vi "Generate Oximetry Plots-Rev1.vi"(10 "Spectral Data":T1={"PDT Amp [v]"=0.0, "RIS Amp [v]"=0.0, "B-Field"=[], "All In-Phase Scan Spectra"=[], "Model Select"=enum."OneCompRISTwoPDT", "Fit Each Scan"=FALSE, "PDT Center [g]"=0.0, "In-Phase Average Spectra"=[], "In-Phase Median Spectra"=[], "Out-Phase Median Spectra"=[], "Out-Phase Average Spectra"=[], "Fit Spectra"=[], "Fit No-Baseline Spectra"=[], "All Out-Phase Scan Spectra"=[], "Baseline Offset Correction"=FALSE, "In-Phase Offset [v]"=0.0, "Out-Phase Offset [v]"=0.0, "Ch2 Input\n(Balance)"=[], "Ch3 Input\n(Phase)"=[], "Ch4 Input\n(AFC)"=[], "Fit Pars"=[], "Fit Pars Errors"=[], "Fit Pars Labels"=[], "Raw Scan DAQ Data"=[], "Bad Scans Indicies"=[], "Good In-Phase Scan Spectra"=[], "Good Out-Phase Scan Spectra"=[], "Bad In-Phase Scan Spectra"=[], "Bad Out-Phase Scan Spectra"=[], "Number of bad scans"=0, "Fit History"=[], "PDT Amp. History/Set [v]"=[], "RIS Amp. History/Set [v]"=[], "RIS Amp. History/Scan [v]"=[], "All Shifted B-Fields"=[], "Good Shifted B-Fields"=[], "Ch5 Input\n(SpO2)"=[], "Ch6 Input\n(BPM)"=[], "Global SNR"=0.0, "Fit Error History"=[], "SNR History"=[]} {"Global SNR" min=0.0; "PDT Center [g]" min=0.0; "RIS Amp [v]" min=0.0; "PDT Amp [v]" min=0.0}, 11 "Measurement Information":T3={"Comments"="", "Directory Input"="", "Data file path"=path "C:/Data/EPR Data", "Scripting File"=path "C:/Data/Configuration Script.csv", "Save Data"=FALSE, "Tooth size (d11) [mm]"=0.0, "Tooth size (d12) [mm]"=0.0, "Tooth size (d21) [mm]"=0.0, "Tooth size (d22) [mm]"=0.0, "Dose of Tooth [Gy]"=0.0, "Safe Shutdown?"=FALSE, "Gases Available"=[], "Database Username"="", "Database Password"="", "Database Login URL"="", "Database Upload URL"="", "Database Success URL"="", "Database XML URL"="", "Database Resonator URL"="", "Session Number"=0, "Set #"=1, "Resonator Operator"="", "Session Type"="", "Tooth/Sample ID"="", "Volunteer ID"="", "Computer Operator"="", "Volunteer Type"="", "Site/Tooth Selection (T8,T9)"="", "Resonator"="", "Measurement Site"="", "Non-standard session?"=FALSE, "EPR DAQ Version"="", "Session Path"=path "C:/Data/EPR Data", "Chosen Applied State"="", "Chosen Initial State"="", "Time of Transition"="", "DAQ Mode"=enum."Engineering", "pO2/Scan [mmHg]"=[], "pO2/Set [mmHg]"=[], "Linewidth (HWHM)/Scan [Gauss]"=[], "Linewidth (HWHM)/Set [Gauss]"=[], "pO2 Conversion"="", "Dose Calibration Cluster"={"Dose Response"={"grand_mean"=0.0292016, "slope"=0.0188720543}, "Dose Correction"={"Sex"=1, "a0"=7.719669421, "a1"=-2.746550736, "a2"=-0.186490355, "a3"=0.041922063, "a4"=-0.849147359, "a5"=0.14330063, "a6"=0.019930219, "A_n"=40.0, "H_n"=10.12, "Dose Correction"=FALSE}, "Dose Reporting"={"Reporting is"=TRUE, "sd_threshold [AU]"=0.06, "sd_model [Gy]"=0.66, "dosimetric_threshold [Gy]"=2.0, "Add intrasession errors is"=FALSE, "Prior Radiation?"=FALSE}}, "OxyChip Slope"=0.0, "OxyChip Intercept"=0.0, "QA Mode"=enum."Select QA Mode", "QA Session?"=FALSE, "Sample Type"=enum."Empty Resonator", "Report pO2/Scan"=FALSE, "Skip End Session Save"=FALSE, "Number of sites"=enum."# Probes", "Recipient Name"="", "Sender Name"="", "Recipient Email"="", "Transition State History"=[], "pO2 Report Times"=[], "Temperature [C]"=0.0, "+Error pO2/Scan [mmHg]"=[], "-Error pO2/Scan [mmHg]"=[], "+Error pO2/Set [mmHg]"=[], "-Error pO2/Set [mmHg]"=[], "Oxy Phase Exclusion Tolerance [rad]"=0.0, "Oxy Center Exclusion Tolerance [%]"=0.0, "Oxy Exclude Unacceptable"=FALSE, "Oxy Unacceptable Estimate Flags"=[], "Save Session PPT"=FALSE, "Flagged Bad Sets"=[]} {"Oxy Center Exclusion Tolerance [%]" format="%#_9g"; "Oxy Phase Exclusion Tolerance [rad]" format="%#_9g"; "Temperature [C]" format="%#_9g"; "OxyChip Intercept" format="%#_9g"; "OxyChip Slope" format="%#_9g"; "Dose Calibration Cluster"."Dose Reporting"."dosimetric_threshold [Gy]" format="%#_9g"; "Dose Calibration Cluster"."Dose Reporting"."sd_model [Gy]" format="%#_9g"; "Dose Calibration Cluster"."Dose Reporting"."sd_threshold [AU]" format="%#_9g"; "Dose Calibration Cluster"."Dose Correction"."H_n" format="%#_9g"; "Dose Calibration Cluster"."Dose Correction"."A_n" format="%#_9g"; "Dose Calibration Cluster"."Dose Correction"."a6" format="%#.9g"; "Dose Calibration Cluster"."Dose Correction"."a5" format="%#.9g"; "Dose Calibration Cluster"."Dose Correction"."a4" format="%#.9g"; "Dose Calibration Cluster"."Dose Correction"."a3" format="%#.9g"; "Dose Calibration Cluster"."Dose Correction"."a2" format="%#.9g"; "Dose Calibration Cluster"."Dose Correction"."a1" format="%#.9g"; "Dose Calibration Cluster"."Dose Correction"."a0" format="%#.9g"; "Dose Calibration Cluster"."Dose Correction"."Sex" items=["Male"=1, "Female"=0]; "Dose Calibration Cluster"."Dose Response"."slope" format="%#_9g"; "Dose Calibration Cluster"."Dose Response"."grand_mean" format="%#_9g"}) -> (0 "error out":errorcluster)   [LabVIEW 2016]
uses:
  Types/Measurement Information.ctl
  Analysis/Dose Calculation and Reporting/Dose Calculation Control.ctl
  Types/Sample Type.ctl
  Types/Spectral Data.ctl
  Types/Fitting Model Selection.ctl
panel:
  out "Spectra Graph\nAutoscaled":cluster{"B-Field":dbl[], "C-Fit":dbl[]}[](graph) caption="Session: 14 || vID#  || March 22, 2017"
  out "Spectra Graph":cluster{"B-Field":dbl[], "C-Fit":dbl[]}[](graph) caption="Session: 14 || vID#  || March 22, 2017"
  # "Session Information"
  # "Oximetric Data and Information"
  # "Email"
  # "Tooth Information"
  # "Database"
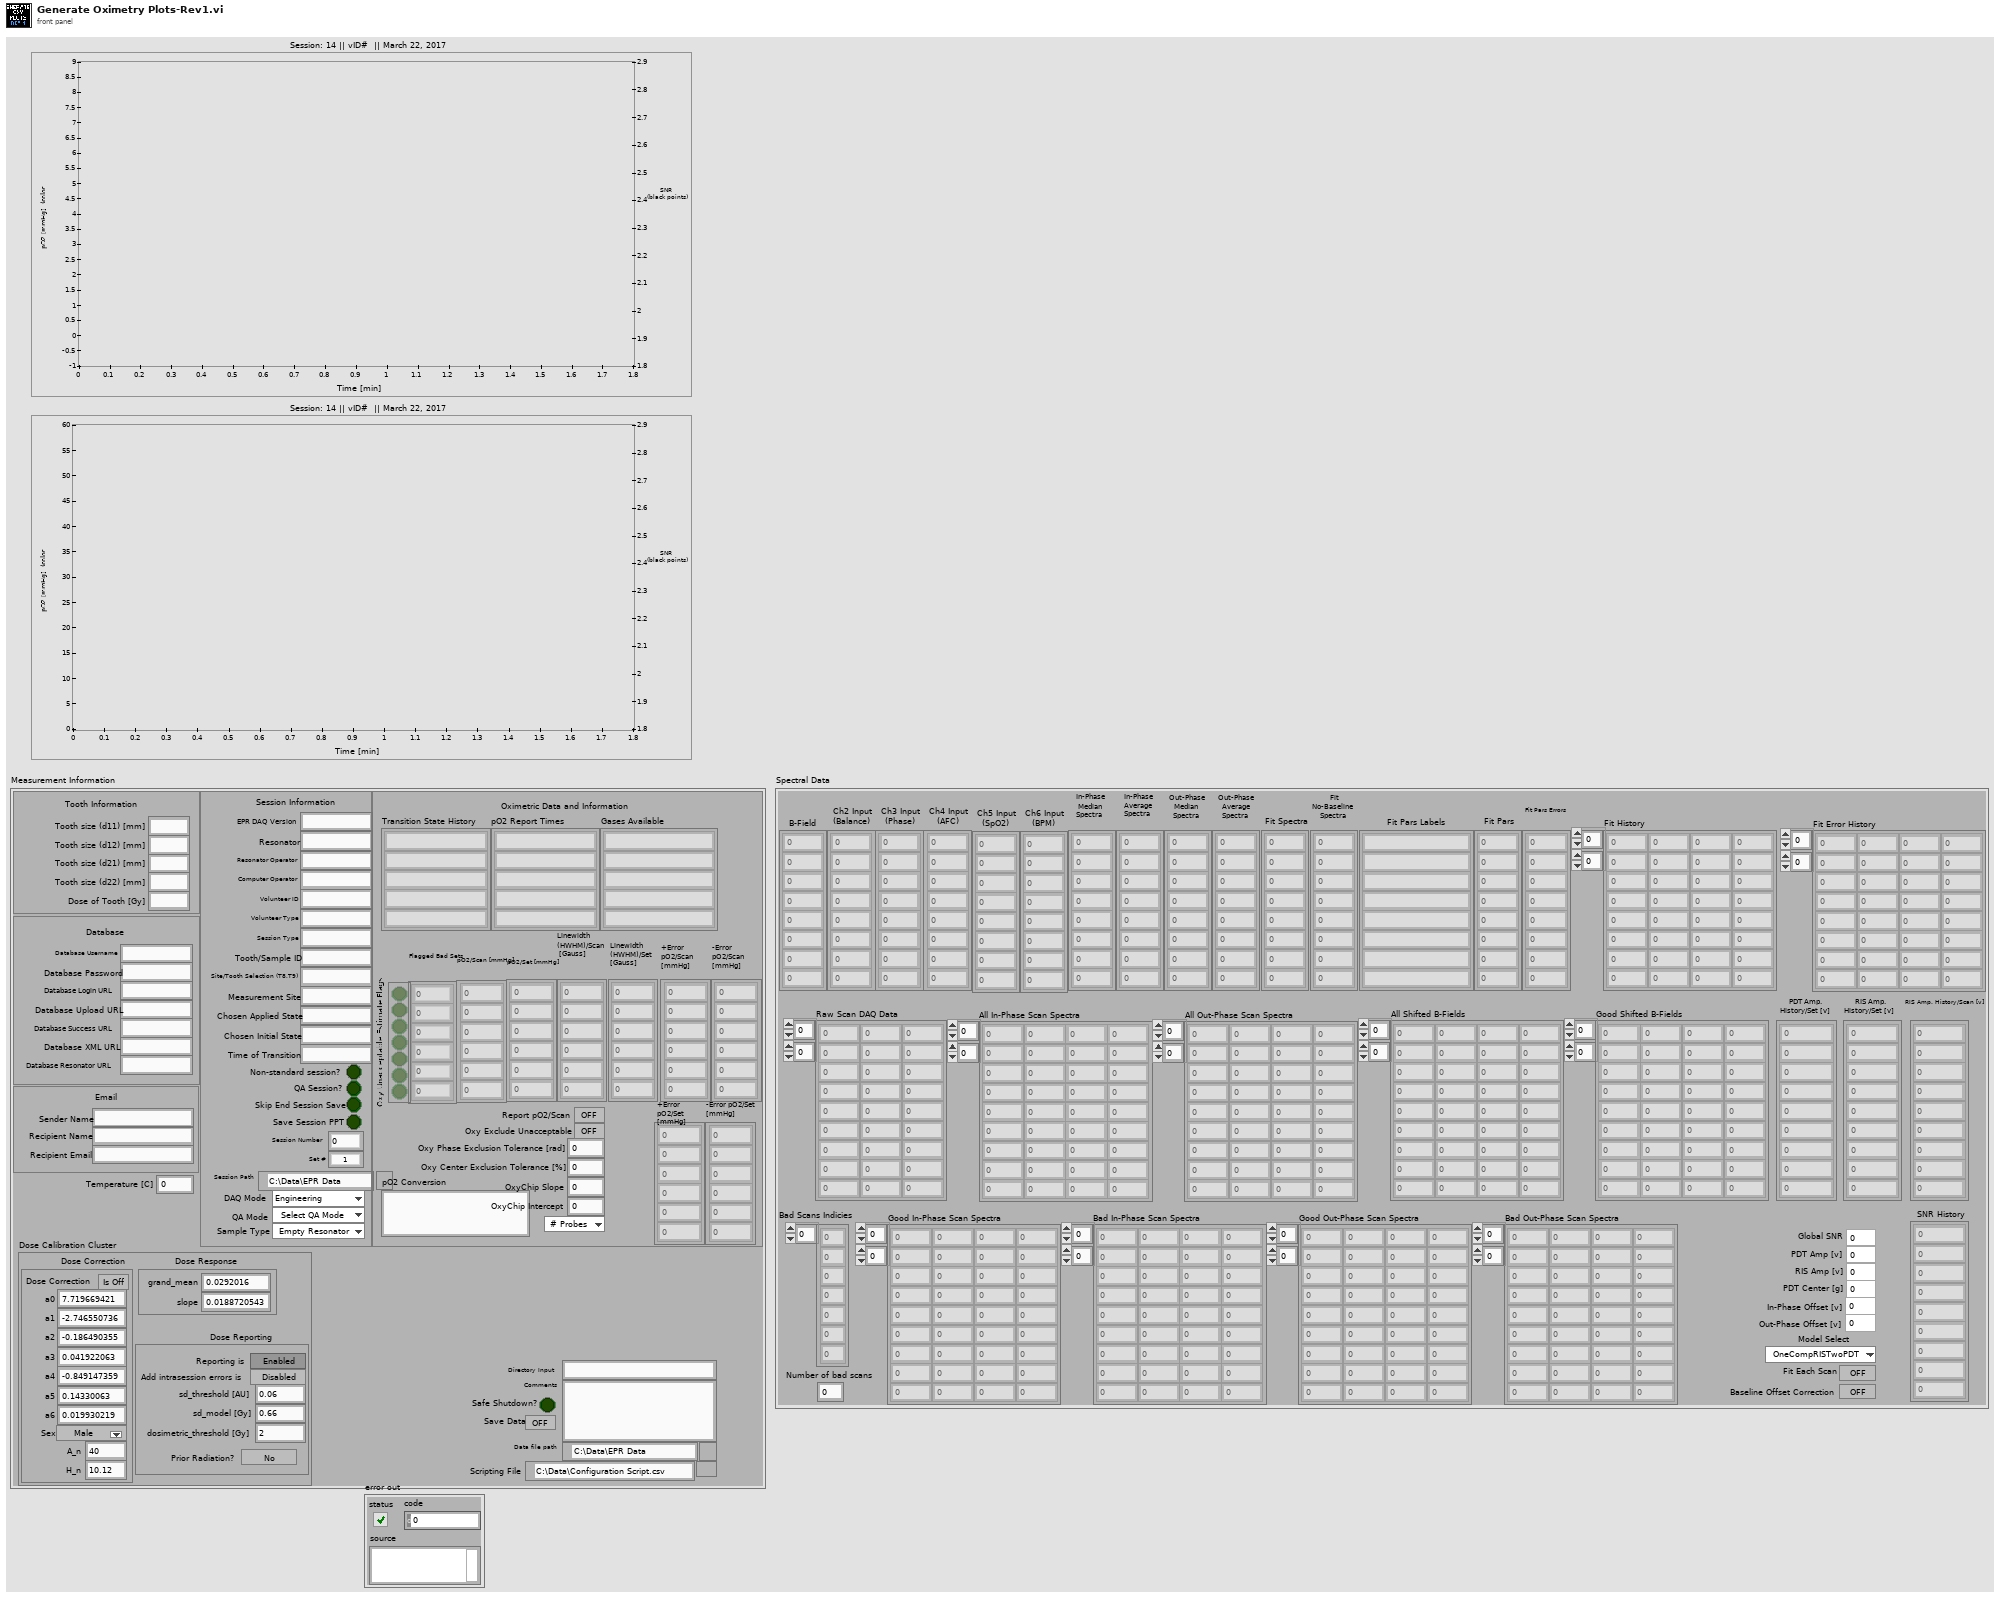
[diagram p1: front panel]
types:
  T1 = typedef "Spectral Data.ctl" = cluster{"PDT Amp [v]":dbl, "RIS Amp [v]":dbl, "B-Field":dbl[], "All In-Phase Scan Spectra":dbl[][], "Model Select":T2, "Fit Each Scan":bool, "PDT Center [g]":dbl, "In-Phase Average Spectra":dbl[], "In-Phase Median Spectra":dbl[], "Out-Phase Median Spectra":dbl[], "Out-Phase Average Spectra":dbl[], "Fit Spectra":dbl[], "Fit No-Baseline Spectra":dbl[], "All Out-Phase Scan Spectra":dbl[][], "Baseline Offset Correction":bool, "In-Phase Offset [v]":dbl, "Out-Phase Offset [v]":dbl, "Ch2 Input\n(Balance)":dbl[], "Ch3 Input\n(Phase)":dbl[], "Ch4 Input\n(AFC)":dbl[], "Fit Pars":dbl[], "Fit Pars Errors":dbl[], "Fit Pars Labels":string[], "Raw Scan DAQ Data":dbl[][], "Bad Scans Indicies":i32[], "Good In-Phase Scan Spectra":dbl[][], "Good Out-Phase Scan Spectra":dbl[][], "Bad In-Phase Scan Spectra":dbl[][], "Bad Out-Phase Scan Spectra":dbl[][], "Number of bad scans":i32, "Fit History":dbl[][], "PDT Amp. History/Set [v]":dbl[], "RIS Amp. History/Set [v]":dbl[], "RIS Amp. History/Scan [v]":dbl[], "All Shifted B-Fields":dbl[][], "Good Shifted B-Fields":dbl[][], "Ch5 Input\n(SpO2)":dbl[], "Ch6 Input\n(BPM)":dbl[], "Global SNR":dbl, "Fit Error History":dbl[][], "SNR History":dbl[]}
  T2 = typedef "Fitting Model Selection.ctl" = enum16{"OneCompRIS", "OneCompRISTwoPDT", "OneCompRISRev", "OneCompRISTwoPDTRev", "LiPc", "TwoLiPc", "ThreeLiPc", "FourLiPc", "PDTCalibration", "CE_Ink", "Printex", "MelaninTwoPDT"}
  T3 = typedef "Measurement Information.ctl" = cluster{"Comments":string, "Directory Input":string, "Data file path":path, "Scripting File":path, "Save Data":bool, "Tooth size (d11) [mm]":dbl, "Tooth size (d12) [mm]":dbl, "Tooth size (d21) [mm]":dbl, "Tooth size (d22) [mm]":dbl, "Dose of Tooth [Gy]":dbl, "Safe Shutdown?":bool, "Gases Available":string[], "Database Username":string, "Database Password":string, "Database Login URL":string, "Database Upload URL":string, "Database Success URL":string, "Database XML URL":string, "Database Resonator URL":string, "Session Number":i32, "Set #":u32, "Resonator Operator":string, "Session Type":string, "Tooth/Sample ID":string, "Volunteer ID":string, "Computer Operator":string, "Volunteer Type":string, "Site/Tooth Selection (T8,T9)":string, "Resonator":string, "Measurement Site":string, "Non-standard session?":bool, "EPR DAQ Version":string, "Session Path":path, "Chosen Applied State":string, "Chosen Initial State":string, "Time of Transition":string, "DAQ Mode":enum16{"Engineering", "Dosimetry", "Oximetry"}, "pO2/Scan [mmHg]":dbl[][], "pO2/Set [mmHg]":dbl[][], "Linewidth (HWHM)/Scan [Gauss]":dbl[][], "Linewidth (HWHM)/Set [Gauss]":dbl[][], "pO2 Conversion":string, "Dose Calibration Cluster":T4, "OxyChip Slope":dbl, "OxyChip Intercept":dbl, "QA Mode":enum16{"Select QA Mode", "QA-Start/End", "QA-Mid", "QA-Weekly", "QA-Eng", "Check Calibration"}, "QA Session?":bool, "Sample Type":T5, "Report pO2/Scan":bool, "Skip End Session Save":bool, "Number of sites":enum16{"# Probes", "1", "2", "3", "4"}, "Recipient Name":string, "Sender Name":string, "Recipient Email":string, "Transition State History":string[], "pO2 Report Times":string[], "Temperature [C]":dbl, "+Error pO2/Scan [mmHg]":dbl[][], "-Error pO2/Scan [mmHg]":dbl[][], "+Error pO2/Set [mmHg]":dbl[][], "-Error pO2/Set [mmHg]":dbl[][], "Oxy Phase Exclusion Tolerance [rad]":dbl, "Oxy Center Exclusion Tolerance [%]":dbl, "Oxy Exclude Unacceptable":bool, "Oxy Unacceptable Estimate Flags":bool[], "Save Session PPT":bool, "Flagged Bad Sets":u32[]}
  T4 = typedef "Dose Calculation Control.ctl" = cluster{"Dose Response":cluster{"grand_mean":dbl, "slope":dbl}, "Dose Correction":cluster{"Sex":u16, "a0":dbl, "a1":dbl, "a2":dbl, "a3":dbl, "a4":dbl, "a5":dbl, "a6":dbl, "A_n":dbl, "H_n":dbl, "Dose Correction":bool}, "Dose Reporting":cluster{"Reporting is":bool, "sd_threshold [AU]":dbl, "sd_model [Gy]":dbl, "dosimetric_threshold [Gy]":dbl, "Add intrasession errors is":bool, "Prior Radiation?":bool}}
  T5 = typedef "Sample Type.ctl" = enum16{"Empty Resonator", "IRS", "BallZero", "Irradiated Tooth", "Non-irradiated Tooth", "OxyChip", "LiPc", "PDT", "India Ink"}
  T6 = cluster{"Good pO2 Estimate Times":dbl[], "Good pO2 Estimates":dbl[]}
  T7 = cluster{"Bad pO2 Estimate Times":dbl[], "Good pO2 Estimates":dbl[]}[]
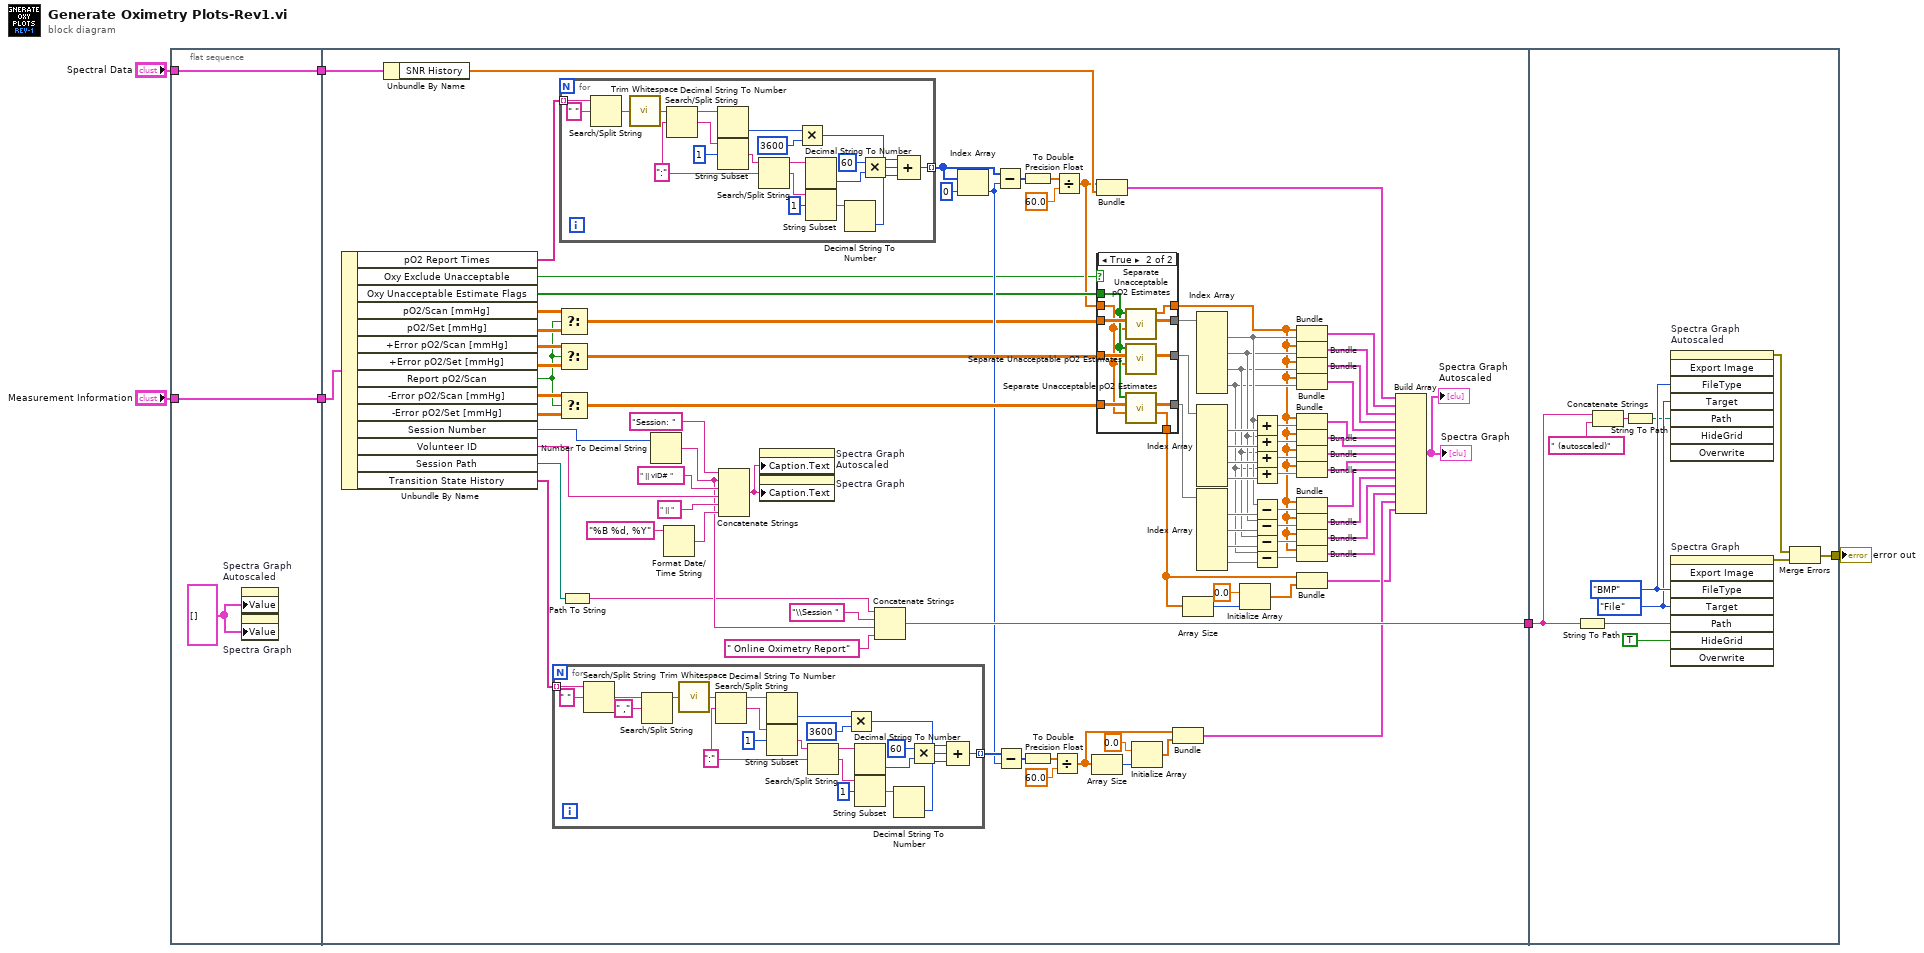
[diagram p0: block diagram]
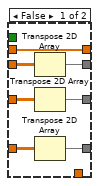
[diagram p2: hidden frame]
diagram:
  n1 = flat-sequence {
    tunnel: "Spectral Data" -> [w8]
    tunnel: "Measurement Information" -> [w9]
    tunnel: [w9] -> w2
    tunnel: [w8] -> w1
    tunnel: [w36] -> w3
    tunnel: w2 -> [w99]
    tunnel: w1 -> [w88]
    tunnel: [w171] -> w4
    tunnel: w3 -> [w170]
    frame #0 {
      w7 = cluster{"B-Field":dbl[], "C-Fit":dbl[]}[] [] ("Spectra Graph\nAutoscaled")
      n2 = property on="Spectra Graph\nAutoscaled" class="XYGraph (strict)"("Value"=w7) -> ()  [unwired: 2 in, 2 out]
      n3 = property on="Spectra Graph" class="XYGraph (strict)"("Value"=w7) -> ()  [unwired: 2 in, 2 out]
    }
    frame #1 {
      n4 = Unbundle By Name(w99) -> ("pO2 Report Times"=w47:string[], "Oxy Exclude Unacceptable"=w15:bool, "Oxy Unacceptable Estimate Flags"=w18:bool[], "pO2/Scan [mmHg]"=w21:dbl[][], "pO2/Set [mmHg]"=w22:dbl[][], "+Error pO2/Scan [mmHg]"=w83:dbl[][], "+Error pO2/Set [mmHg]"=w82:dbl[][], "Report pO2/Scan"=w19:bool, "-Error pO2/Scan [mmHg]"=w81:dbl[][], "-Error pO2/Set [mmHg]"=w80:dbl[][], "Session Number"=w85:i32, "Volunteer ID"=w84:string, "Session Path"=w39:path, "Transition State History"=w34:string[])
      n5 = Unbundle By Name(w88) -> ("SNR History"=w87:dbl[])
      n6 = for {
        tunnel: w34 -> [w120] mode=indexing
        tunnel: [w121] -> w33 mode=indexing
        w133 = ":" ("search string/char (-)")
        n7 = Search/Split String(string=w120, search string/char (-)=" ") -> (match + rest of string=w118:string)  [unwired: 1 in, 2 out]
        n8 = Search/Split String(string=w118, search string/char (-)=" ,") -> (substring before match=w117:string)  [unwired: 1 in, 2 out]
        n9 = call <vilib>:"Trim Whitespace.vi"("string"=w117) -> ("trimmed string"=w138:string)  [unwired: 1 in]
        n10 = Search/Split String(string=w138, search string/char (-)=w133) -> (substring before match=w137:string, match + rest of string=w136:string)  [unwired: 1 in, 1 out]
        n11 = Decimal String To Number(string=w137) -> (number=w128:i32)  [unwired: 2 in, 1 out]
        n12 = String Subset(string=w136, offset (0)=1) -> (substring=w134:string)  [unwired: 1 in]
        n13 = Search/Split String(string=w134, search string/char (-)=w133) -> (substring before match=w132:string, match + rest of string=w130:string)  [unwired: 1 in, 1 out]
        n14 = Multiply(x=w128, y=3600) -> (x*y=w123:i32)
        n15 = Decimal String To Number(string=w132) -> (number=w125:i32)  [unwired: 2 in, 1 out]
        n16 = String Subset(string=w130, offset (0)=1) -> (substring=w129:string)  [unwired: 1 in]
        n17 = Decimal String To Number(string=w129) -> (number=w122:i32)  [unwired: 2 in, 1 out]
        n18 = Multiply(x=60, y=w125) -> (x*y=w124:i32)
        n19 = Compound Arithmetic op=ADD(w123, w124, w122) -> (w121:i32)
      }
      n20 = Select(t=w21, s=w19, f=w22) -> (s? t:f=w20:dbl[][])
      n21 = Select(t=w83, s=w19, f=w82) -> (s? t:f=w79:dbl[][])
      n22 = Select(t=w81, s=w19, f=w80) -> (s? t:f=w78:dbl[][])
      n23 = for {
        tunnel: w47 -> [w140] mode=indexing
        tunnel: [w141] -> w32 mode=indexing
        w153 = ":" ("search string/char (-)")
        n24 = Search/Split String(string=w140, search string/char (-)=" ") -> (match + rest of string=w159:string)  [unwired: 1 in, 2 out]
        n25 = call <vilib>:"Trim Whitespace.vi"("string"=w159) -> ("trimmed string"=w158:string)  [unwired: 1 in]
        n26 = Search/Split String(string=w158, search string/char (-)=w153) -> (substring before match=w157:string, match + rest of string=w156:string)  [unwired: 1 in, 1 out]
        n27 = Decimal String To Number(string=w157) -> (number=w148:i32)  [unwired: 2 in, 1 out]
        n28 = String Subset(string=w156, offset (0)=1) -> (substring=w154:string)  [unwired: 1 in]
        n29 = Search/Split String(string=w154, search string/char (-)=w153) -> (substring before match=w152:string, match + rest of string=w150:string)  [unwired: 1 in, 1 out]
        n30 = Multiply(x=w148, y=3600) -> (x*y=w143:i32)
        n31 = Decimal String To Number(string=w152) -> (number=w145:i32)  [unwired: 2 in, 1 out]
        n32 = String Subset(string=w150, offset (0)=1) -> (substring=w149:string)  [unwired: 1 in]
        n33 = Decimal String To Number(string=w149) -> (number=w142:i32)  [unwired: 2 in, 1 out]
        n34 = Multiply(x=60, y=w145) -> (x*y=w144:i32)
        n35 = Compound Arithmetic op=ADD(w143, w144, w142) -> (w141:i32)
      }
      n36 = Path To String(path=w39) -> (string=w38:string)
      n37 = Number To Decimal String(number=w85) -> (decimal integer string=w41:string)  [unwired: 1 in]
      n38 = Format Date/Time String(time format string (%c)="%B %d, %Y") -> (date/time string=w94:string)  [unwired: 2 in]
      n39 = Concatenate Strings("Session: " ("string"), w41, " || vID# " ("string"), w84, " || " ("string"), w94) -> (w35:string)
      n40 = property on="Spectra Graph\nAutoscaled" class="XYGraph (strict)"("Caption.Text"=w35) -> ()  [unwired: 2 in, 2 out]
      n41 = property on="Spectra Graph" class="XYGraph (strict)"("Caption.Text"=w35) -> ()  [unwired: 2 in, 2 out]
      n42 = Concatenate Strings(w38, "\\Session " ("string"), w41, " Online Oximetry Report" ("string")) -> (w36:string)
      n43 = Index Array(array=w32, index=0) -> (element=w28:i32)
      n44 = Subtract(x=w32, y=w28) -> (x-y=w45:i32[])
      n45 = Subtract(x=w33, y=w28) -> (x-y=w31:i32[])
      n46 = To Double Precision Float(number=w45) -> (double precision float=w43:dbl[])
      n47 = To Double Precision Float(number=w31) -> (double precision float=w30:dbl[])
      n48 = Divide(x=w30, y=60.0 ("index")) -> (x/y=w24:dbl[])
      n49 = Divide(x=w43, y=60.0 ("index")) -> (x/y=w17:dbl[])
      n50 = Array Size(array=w24) -> (size(s)=w26:i32)
      n51 = Bundle(w17, "SNR History"=w87) -> (w86:cluster{dbl[], "SNR History":dbl[]})  [unwired: 1 in]
      n52 = case shown="True" w15 {
        tunnel: [w106 w110] -> w89
        tunnel: w79 -> [w105 w115]
        tunnel: w78 -> [w104 w113]
        tunnel: [w103 w109] -> w77
        tunnel: [w102 w108] -> w76
        tunnel: w20 -> [w101 w116]
        tunnel: w18 -> [_ w114]
        tunnel: w17 -> [w100 w112]
        tunnel: [w100 w111] -> w16
        tunnel: [_ w107] -> w11
        frame False {
          n53 = Transpose 2D Array(2D array=w101) -> (transposed array=w106:dbl[][])
          n54 = Transpose 2D Array(2D array=w105) -> (transposed array=w103:dbl[][])
          n55 = Transpose 2D Array(2D array=w104) -> (transposed array=w102:dbl[][])
        }
        frame True {
          n56 = call "Separate Unacceptable pO2 Estimates.vi"("All Times"=w112, "All pO2 Estimates"=w116, "Oxy Unacceptable Estimate Flags"=w114) -> ("Good pO2 Estimates"=w110:dbl[][], "Good pO2 Estimate Times"=w111:dbl[])  [unwired: 5 in, 2 out]
          n57 = call "Separate Unacceptable pO2 Estimates.vi"("All Times"=w112, "All pO2 Estimates"=w115, "Oxy Unacceptable Estimate Flags"=w114) -> ("Good pO2 Estimates"=w109:dbl[][])  [unwired: 5 in, 3 out]
          n58 = call "Separate Unacceptable pO2 Estimates.vi"("All Times"=w112, "All pO2 Estimates"=w113, "Oxy Unacceptable Estimate Flags"=w114) -> ("Bad pO2 Estimate Times"=w107:dbl[], "Good pO2 Estimates"=w108:dbl[][])  [unwired: 5 in, 2 out]
        }
      }
      n59 = Initialize Array(0.0 ("element"), w26) -> (w23:dbl[])
      n60 = Bundle(w24, w23) -> (w25:cluster{dbl[], dbl[]})  [unwired: 1 in]
      n61 = Array Size(array=w11) -> (size(s)=w13:i32)
      n62 = Index Array(array=w89) -> (element #1=w55:dbl[], element #2=w54:dbl[], element #3=w53:dbl[], element #4=w52:dbl[])  [unwired: 8 in]
      n63 = Index Array(array=w77) -> (element #1=w67:dbl[], element #2=w66:dbl[], element #3=w65:dbl[], element #4=w64:dbl[])  [unwired: 8 in]
      n64 = Index Array(array=w76) -> (element #1=w59:dbl[], element #2=w58:dbl[], element #3=w57:dbl[], element #4=w56:dbl[])  [unwired: 8 in]
      n65 = Initialize Array(0.0 ("element"), w13) -> (w10:dbl[])
      n66 = Add(x=w55, y=w67) -> (x+y=w63:dbl[])
      n67 = Add(x=w54, y=w66) -> (x+y=w62:dbl[])
      n68 = Add(x=w53, y=w65) -> (x+y=w61:dbl[])
      n69 = Add(x=w52, y=w64) -> (x+y=w60:dbl[])
      n70 = Subtract(x=w55, y=w59) -> (x-y=w51:dbl[])
      n71 = Subtract(x=w54, y=w58) -> (x-y=w50:dbl[])
      n72 = Subtract(x=w53, y=w57) -> (x-y=w49:dbl[])
      n73 = Subtract(x=w52, y=w56) -> (x-y=w48:dbl[])
      n74 = Bundle("Good pO2 Estimate Times"=w16, "Good pO2 Estimates"=w55) -> (w93:T6)  [unwired: 1 in]
      n75 = Bundle("Good pO2 Estimate Times"=w16, "Good pO2 Estimates"=w54) -> (w92:T6)  [unwired: 1 in]
      n76 = Bundle("Good pO2 Estimate Times"=w16, "Good pO2 Estimates"=w53) -> (w91:T6)  [unwired: 1 in]
      n77 = Bundle("Good pO2 Estimate Times"=w16, "Good pO2 Estimates"=w52) -> (w90:T6)  [unwired: 1 in]
      n78 = Bundle("Good pO2 Estimate Times"=w16, w63) -> (w75:cluster{"Good pO2 Estimate Times":dbl[], dbl[]})  [unwired: 1 in]
      n79 = Bundle("Good pO2 Estimate Times"=w16, w62) -> (w74:cluster{"Good pO2 Estimate Times":dbl[], dbl[]})  [unwired: 1 in]
      n80 = Bundle("Good pO2 Estimate Times"=w16, w61) -> (w73:cluster{"Good pO2 Estimate Times":dbl[], dbl[]})  [unwired: 1 in]
      n81 = Bundle("Good pO2 Estimate Times"=w16, w60) -> (w72:cluster{"Good pO2 Estimate Times":dbl[], dbl[]})  [unwired: 1 in]
      n82 = Bundle("Good pO2 Estimate Times"=w16, w51) -> (w71:cluster{"Good pO2 Estimate Times":dbl[], dbl[]})  [unwired: 1 in]
      n83 = Bundle("Good pO2 Estimate Times"=w16, w50) -> (w70:cluster{"Good pO2 Estimate Times":dbl[], dbl[]})  [unwired: 1 in]
      n84 = Bundle("Good pO2 Estimate Times"=w16, w49) -> (w69:cluster{"Good pO2 Estimate Times":dbl[], dbl[]})  [unwired: 1 in]
      n85 = Bundle("Good pO2 Estimate Times"=w16, w48) -> (w68:cluster{"Good pO2 Estimate Times":dbl[], dbl[]})  [unwired: 1 in]
      n86 = Bundle("Bad pO2 Estimate Times"=w11, w10) -> (w14:cluster{"Bad pO2 Estimate Times":dbl[], dbl[]})  [unwired: 1 in]
      n87 = Build Array(w86, w93, w92, w91, w90, w75, w74, w73, w72, w71, w70, w69, w68, w25, w14) -> (→"Spectra Graph" →"Spectra Graph\nAutoscaled":T7)
    }
    frame #2 {
      w167 = enum32{"File", "Clipboard"}."File" ("Target")
      w168 = enum32{"BMP", "EPS", "EMF", "PICT"}."BMP" ("File Type")
      n88 = String To Path(string=w170) -> (path=w164:path)
      n89 = Concatenate Strings(w170, " (autoscaled)" ("string")) -> (w161:string)
      n90 = String To Path(string=w161) -> (path=w163:path)
      n91 = invoke on="Spectra Graph\nAutoscaled" class="XYGraph (strict)" method="Export Image"("FileType"=w168, "Target"=w167, "Path"=w163) -> (error out=w165:errorcluster)  [unwired: 5 in, 7 out]
      n92 = invoke on="Spectra Graph" class="XYGraph (strict)" method="Export Image"("FileType"=w168, "Target"=w167, "Path"=w164, "HideGrid"=TRUE ("Hide Grid")) -> (error out=w166:errorcluster)  [unwired: 4 in, 7 out]
      n93 = Merge Errors(w165, w166) -> (w171:errorcluster)
    }
  }
  "error out" <- w4
